vi "MediaPlayer_Create.vi"(0 "reference in":refnum<class "MediaPlayer.lvclass">, 5 "Music List":path[](array[path]), 7 "Device ID":u32, 11 "Error In":errorcluster) -> (4 "reference out":refnum<class "MediaPlayer.lvclass">, 15 "Error Out":errorcluster)   [LabVIEW 2024, in "MediaPlayer.lvclass"]
uses:
  MediaPlayer.lvclass
  MediaPlayer.lvclass/MediaPlayer.ctl
panel:
  # "Connector Pane"
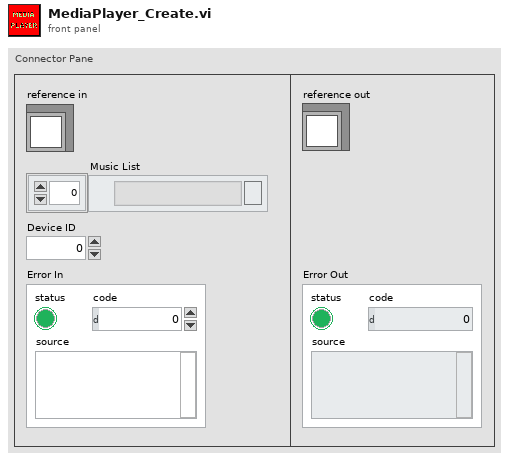
[diagram p1: front panel]
types:
  T1 = typedef "MediaPlayer.lvclass/ObjectAttributes.ctl" = cluster{"MediaPlayerData":T2, "Current Info":cluster{"Duration":dbl, "Name":string, "Is playing?":bool}}
  T2 = typedef "MediaPlayer.lvclass/MediaPlayer Data.ctl" = cluster{"Music List":path[], "Current Music Index":u16, "Song Handler":T3, "Device ID":u32}
  T3 = typedef "Sound Output Task ID.ctl" = u32
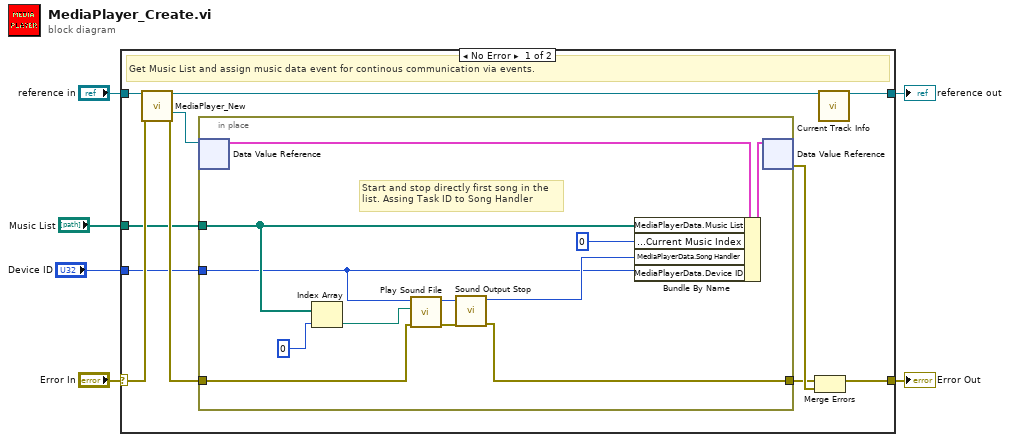
[diagram p0: block diagram]
diagram:
  n1 = case shown="No Error" "Error In" {
    selector: "Error In" -> [w16 w31]
    tunnel: [w11 w31] -> w5
    tunnel: "reference in" -> [w17 w30]
    tunnel: [w7 w30] -> w3
    tunnel: "Music List" -> [w10 _]
    tunnel: "Device ID" -> [w9 _]
    frame No Error {
      # "Get Music List and assign music data event for continous communication via events."
      n2 = call "MediaPlayer_New.vi"("reference in"=w17, "Error In"=w16) -> ("reference out"=w8:refnum<class "MediaPlayer.lvclass">, "DVRRefOut"=w14:refnum<data-value>, "Error Out"=w13:errorcluster)  [unwired: 10 in, 1 out]
      n3 = in-place {
        in-place-border: w13 -> [w21]
        in-place-border: [w20] -> w12
        in-place-border: w10 -> [w23]
        in-place-border: w9 -> [w19]
        # "Start and stop directly first song in the\nlist. Assing Task ID to Song Handler"
        n4 = in-place-dvr #1(w14) -> (w28:T1)  [unwired: 1 out]
        n5 = Index Array(array=w23, index=0) -> (element=w24:path)
        n6 = call <vilib>:"Play Sound File.vi"("error in (no error)"=w21, "path"=w24, "device ID"=w19) -> ("error out"=w26:errorcluster, "task ID"=w25:T3)  [unwired: 7 in]
        n7 = call <vilib>:"Sound Output Stop.vi"("error in (no error)"=w26, "task ID"=w25) -> ("error out"=w20:errorcluster, "task ID out"=w22:T3)  [unwired: 8 in]
        n8 = Bundle By Name(cluster=w28, "MediaPlayerData.Music List"=w23, "MediaPlayerData.Current Music Index"=u16 0 ("Current Music"), "MediaPlayerData.Song Handler"=w22, "MediaPlayerData.Device ID"=w19) -> (w29:T1)
        n9 = in-place-dvr #1(w29) -> (w15:errorcluster)  [unwired: 1 out]
      }
      n10 = Merge Errors(w12, w15) -> (w11:errorcluster)
      n11 = call-dynamic "Current Track Info.vi"("reference in"=w8) -> ("reference out"=w7:refnum<class "MediaPlayer.lvclass">)  [unwired: 13 in, 1 out]
    }
    frame Error {
      # "VI-TechBaseTemplate_Simple_4x4x4"
    }
  }
  "Error Out" <- w5
  "reference out" <- w3
